vi "Comparision.vi"(10 "IN":dbl, 11 "ENG":dbl) -> (3 "ENG OUT":dbl)   [LabVIEW 2020]
doc: "This SubVi is optional to use: if, by any means the proton would exeed the speed which it should never have, its velocity is decerasing to begining."
uses:
  Global variables.vi
panel:
  # "This SubVi resets energy to base level after end of animation"
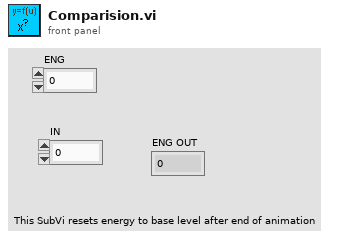
[diagram p1: front panel]
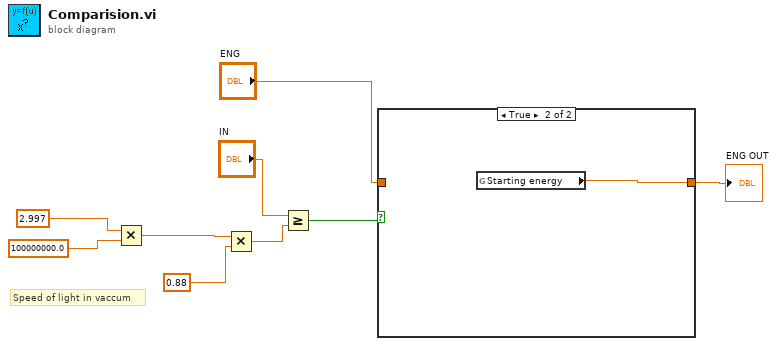
[diagram p0: block diagram]
diagram:
  # "Speed of light in vaccum"
  n1 = Multiply(x=2.997, y=100000000.0) -> (x*y=w2:dbl)
  n2 = Multiply(x=w2, y=0.88) -> (x*y=w9:dbl)
  n3 = Greater Or Equal?(x="IN", y=w9) -> (x >= y?=w7:bool)
  n4 = case shown="True" w7 {
    tunnel: [w10 w11] -> w6
    tunnel: "ENG" -> [w10 _]
    frame False {
    }
    frame True {
      n5 = global read "Global variables.vi" "Starting energy"() -> (w11:dbl)
    }
  }
  "ENG OUT" <- w6
